vi "misurazione_distanza(subVI).vi"(7 "Image Dst":T1, 8 "error in (no error)":errorcluster, 9 "punto 1":i32=1, 10 "punto 0":i32, 11 "Image SRC":T1) -> (0 "error out":errorcluster)   [LabVIEW 2020]
doc: "Fornisce in uscita la distanza tra due particelle sia in real word se l'immagine è stata calibrata che come distanza tra pixel."
uses:
  <vilib>/vision/Image Controls.llb/IMAQ Image.ctl
  <vilib>/vision/NI_Vision_Development_Module.lvlib
panel:
  out "Image 2":T1(plugin-control)
  in  "Pixel":bool
  out "Image":T1(plugin-control)
  in  "stop":bool
  # "Real-Word"
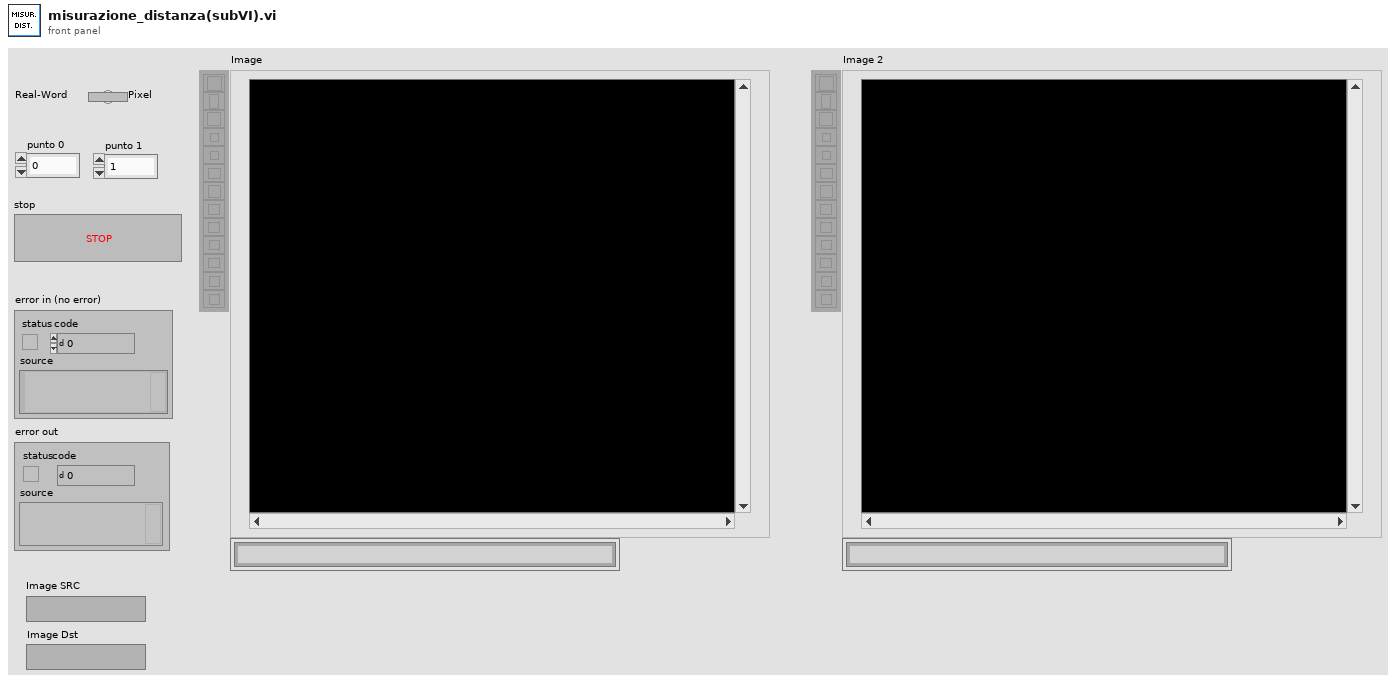
[diagram p1: front panel]
types:
  T1 = typedef "IMAQ Image.ctl" = refnum<image>
  T2 = cluster{"Desired Font (Application)":enum16{"User-specified Font", "Application Font", "System Font", "Dialog Font"}, "[User-specified Font]":cluster{"Font Name":string, "Size":i16, "Strikeout?":bool, "Italic?":bool, "Underline?":bool, "Outline?":bool, "Shadow?":bool, "Bold?":bool, "Rotation Angle":dbl}, "Horizontal Alignment":i16, "Vertical Alignment":i16}
  T3 = cluster{"Area":dbl, "Number of Holes":dbl, "Bounding Rect":cluster{"Left":dbl, "Top":dbl, "Right":dbl, "Bottom":dbl}, "Center of Mass":cluster{"X":dbl, "Y":dbl}, "Orientation":dbl, "Dimensions":cluster{"Width":dbl, "Height":dbl}}[]
  T4 = cluster{"Area":dbl, "Number of Holes":dbl, "Bounding Rect":cluster{"Left":dbl, "Top":dbl, "Right":dbl, "Bottom":dbl}, "Center of Mass":cluster{"X":dbl, "Y":dbl}, "Orientation":dbl, "Dimensions":cluster{"Width":dbl, "Height":dbl}}
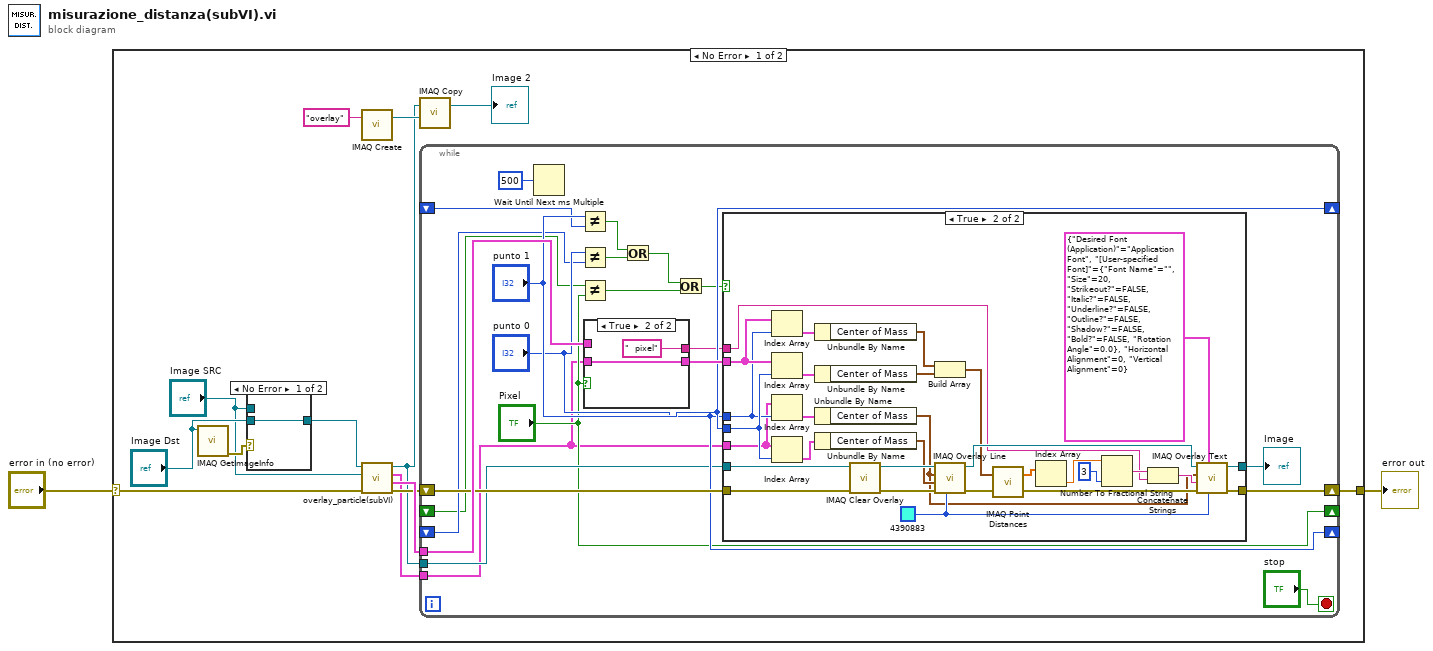
[diagram p0: block diagram]
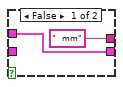
[diagram p4: hidden frame]
diagram:
  n1 = case shown="No Error" "error in (no error)" {
    selector: "error in (no error)" -> [w11 w75]
    tunnel: [w15 w75] -> w2
    frame No Error {
      n2 = call "IMAQ GetImageInfo"("Image"="Image Dst") -> ("error out"=w14:errorcluster)  [unwired: 3 in, 7 out]
      n3 = case shown="No Error" w14 {
        tunnel: "Image Dst" -> [w16 _]
        tunnel: [w16 w17] -> w4
        tunnel: "Image SRC" -> [_ w17]
        frame No Error {
        }
        frame Error {
        }
      }
      n4 = call "IMAQ Create"("Image Name"="overlay") -> ("New Image"=w8:T1)  [unwired: 4 in, 1 out]
      n5 = call "overlay_particle(subVI).vi"("error in (no error)"=w11, "image source"="Image SRC", "image dst"=w4) -> ("error out"=w10:errorcluster, "Particle Reports (Real-World)"=w12:T3, "Particle Reports (Pixels)"=w3:T3, "image Out"=w6:T1)  [unwired: 4 in, 1 out]
      n6 = call "IMAQ Copy"("Image Dst"=w8, "Image Src"=w6) -> ("Image Dst Out"=→"Image 2":T1)  [unwired: 4 in, 1 out]
      n7 = while {
        shift-right: [w36] -> w15
        shift-left: w10 -> [w35]
        tunnel: w12 -> [w38]
        tunnel: w6 -> [w25]
        shift-right: ["punto 1"] -> _
        shift-left: _ -> [w31]
        shift-right: ["punto 0"] -> _
        shift-left: _ -> [w29]
        shift-right: ["Pixel"] -> _
        shift-left: _ -> [w22]
        tunnel: w3 -> [w18]
        stop <- "stop" stop-if-true
        n8 = Wait Until Next ms Multiple(millisecond multiple=u32 500) -> ()  [unwired: 1 out]
        n9 = Not Equal?(x="punto 1", y=w31) -> (x != y?=w28:bool)
        n10 = Not Equal?(x="punto 0", y=w29) -> (x != y?=w27:bool)
        n11 = Not Equal?(x=w22, y="Pixel") -> (x != y?=w20:bool)
        n12 = case shown="True" "Pixel" {
          tunnel: [w72 w73] -> w37
          tunnel: w38 -> [w72 _]
          tunnel: ["  mm" "  pixel"] -> w24
          tunnel: w18 -> [_ w73]
          frame False {
          }
          frame True {
          }
        }
        n13 = Or(x=w28, y=w27) -> (x .or. y?=w23:bool)
        n14 = Or(x=w23, y=w20) -> (x .or. y?=w19:bool)
        n15 = case shown="True" w19 {
          tunnel: w37 -> [_ w56]
          tunnel: w25 -> [w39 w51]
          tunnel: [w40 w63] -> w36
          tunnel: w35 -> [w40 w49]
          tunnel: "punto 1" -> [_ w55]
          tunnel: "punto 0" -> [_ w54]
          tunnel: [w39 w62] -> w26
          tunnel: w24 -> [_ w47]
          tunnel: w18 -> [_ w43]
          frame False {
          }
          frame True {
            w65 = u32 4390883 ("Color")
            n16 = Index Array(array=w56, index=w54) -> (element=w61:T4)
            n17 = Index Array(array=w56, index=w55) -> (element=w60:T4)
            n18 = Index Array(array=w43, index=w54) -> (element=w44:T4)
            n19 = Index Array(array=w43, index=w55) -> (element=w42:T4)
            n20 = Unbundle By Name(w61) -> ("Center of Mass"=w59:cluster{"X":dbl, "Y":dbl})
            n21 = Unbundle By Name(w60) -> ("Center of Mass"=w58:cluster{"X":dbl, "Y":dbl})
            n22 = Unbundle By Name(w44) -> ("Center of Mass"=w41:cluster{"X":dbl, "Y":dbl})
            n23 = Unbundle By Name(w42) -> ("Center of Mass"=w45:cluster{"X":dbl, "Y":dbl})
            n24 = call "IMAQ Clear Overlay"("error in (no error)"=w49, "Image"=w51) -> ("error out"=w48:errorcluster, "Image Out"=w50:T1)  [unwired: 8 in]
            n25 = Build Array(w59, w58) -> (w57:cluster{"X":dbl, "Y":dbl}[])
            n26 = call "IMAQ Overlay Line"("Color"=w65, "error in (no error)"=w48, "End Point"=w45, "Start Point"=w41, "Image"=w50) -> ("error out"=w66:errorcluster, "Image Out"=w64:T1)  [unwired: 5 in]
            n27 = call "IMAQ Point Distances"("Points"=w57, "error in (no error)"=w66) -> ("Distances"=w67:sgl[], "error out"=w69:errorcluster)  [unwired: 3 in]
            n28 = Index Array(array=w67) -> (element=w68:sgl)  [unwired: 1 in]
            n29 = Number To Fractional String(number=w68, precision (6)=i16 3) -> (F-format string=w53:string)  [unwired: 2 in]
            n30 = Concatenate Strings(w53, w47) -> (w70:string)
            n31 = call "IMAQ Overlay Text"("Text Color (black)"=w65, "Font, Size & Style"=T2 {"Desired Font (Application)"=enum."Application Font", "[User-specified Font]"={"Font Name"="", "Size"=20, "Strikeout?"=FALSE, "Italic?"=FALSE, "Underline?"=FALSE, "Outline?"=FALSE, "Shadow?"=FALSE, "Bold?"=FALSE, "Rotation Angle"=0.0}, "Horizontal Alignment"=0, "Vertical Alignment"=0}, "error in (no error)"=w69, "String"=w70, "Origin"=w41, "Image"=w64) -> ("error out"=w63:errorcluster, "Image Out"=w62:T1)  [unwired: 4 in]
          }
        }
        "Image" <- w26
      }
    }
    frame Error {
    }
  }
  "error out" <- w2
